vi "Andres  Decoder 3-to-8      Complete.vi"() -> ()   [LabVIEW 2013]
panel:
  out "Boolean 7":bool
  out "Boolean 6":bool
  out "Boolean 5":bool
  out "Boolean 4":bool
  out "Boolean 3":bool
  out "Boolean 2":bool
  out "Boolean 1":bool
  out "Boolean 0":bool
  in  "Digital 2":bool
  in  "Digital 0":bool
  in  "Digital 1":bool
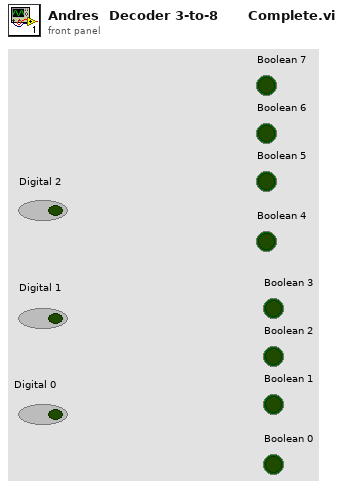
[diagram p1: front panel]
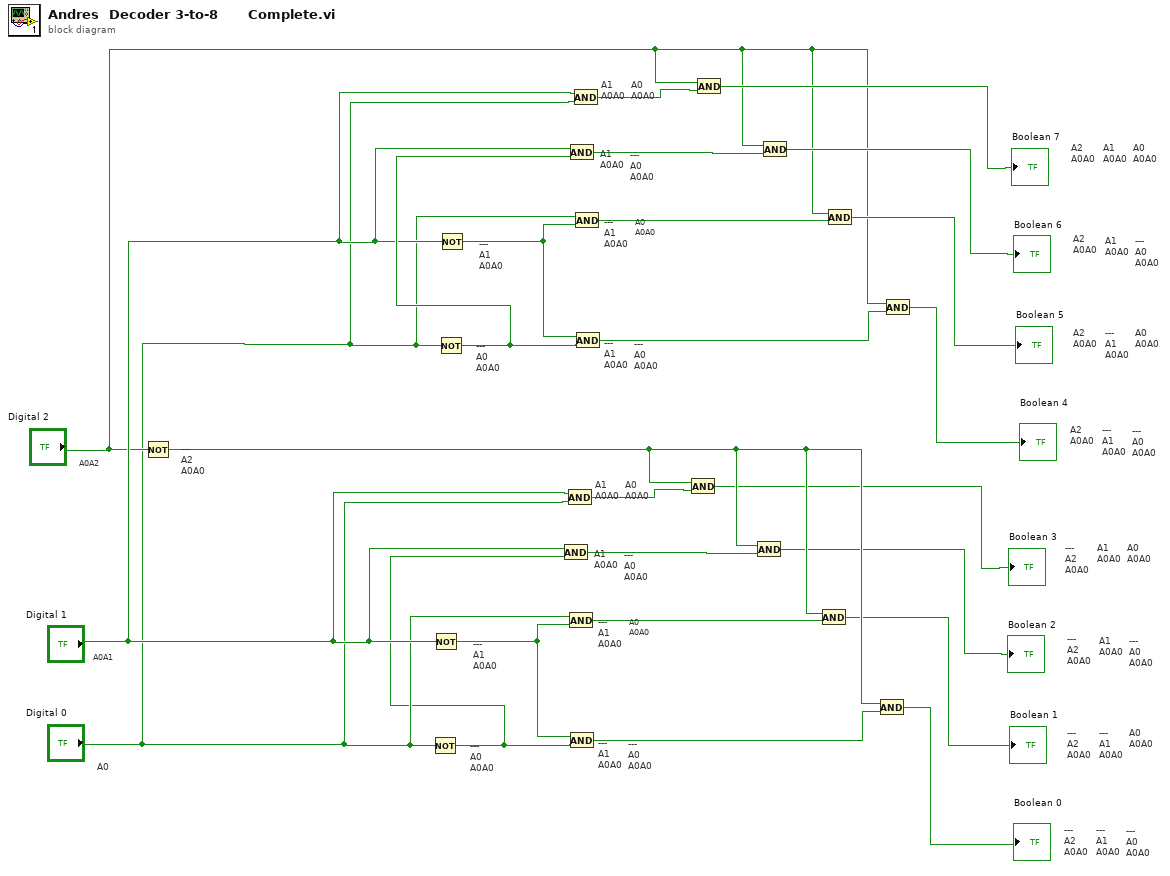
[diagram p0: block diagram]
diagram:
  # "A1\nA0A0"
  # "A0\nA0A0"
  # "---\nA2\nA0A0"
  # "A1\nA0A0"
  # "A0\nA0A0"
  # "A1\nA0A0"
  # "---\nA0\nA0A0"
  # "---\nA2\nA0A0"
  # "A1\nA0A0"
  # "---\nA0\nA0A0"
  # "---\nA1\nA0A0"
  # "A0\nA0A0"
  # "---\nA2\nA0A0"
  # "---\nA1\nA0A0"
  # "A0\nA0A0"
  # "---\nA2\nA0A0"
  # "---\nA1\nA0A0"
  # "---\nA0\nA0A0"
  # "---\nA1\nA0A0"
  # "---\nA0\nA0A0"
  # "---\nA1\nA0A0"
  # "---\nA0\nA0A0"
  # "A1\nA0A0"
  # "A0\nA0A0"
  # "A2\nA0A0"
  # "A1\nA0A0"
  # "A0\nA0A0"
  # "A1\nA0A0"
  # "---\nA0\nA0A0"
  # "A2\nA0A0"
  # "A1\nA0A0"
  # "---\nA0\nA0A0"
  # "---\nA1\nA0A0"
  # "A0\nA0A0"
  # "A2\nA0A0"
  # "---\nA1\nA0A0"
  # "A0\nA0A0"
  # "A2\nA0A0"
  # "---\nA1\nA0A0"
  # "---\nA0\nA0A0"
  # "---\nA1\nA0A0"
  # "---\nA0\nA0A0"
  # "---\nA1\nA0A0"
  # "---\nA0\nA0A0"
  # "A0A1"
  # "A0"
  # "---\nA2\nA0A0"
  # "A0A2"
  n1 = Not(x="Digital 2") -> (.not. x?=w24:bool)
  n2 = Not(x="Digital 0") -> (.not. x?=w5:bool)
  n3 = Not(x="Digital 1") -> (.not. x?=w8:bool)
  n4 = Not(x="Digital 0") -> (.not. x?=w19:bool)
  n5 = Not(x="Digital 1") -> (.not. x?=w22:bool)
  n6 = And(x="Digital 1", y=w5) -> (x .and. y?=w4:bool)
  n7 = And(x="Digital 1", y="Digital 0") -> (x .and. y?=w2:bool)
  n8 = And(x="Digital 0", y=w8) -> (x .and. y?=w7:bool)
  n9 = And(x="Digital 1", y=w19) -> (x .and. y?=w18:bool)
  n10 = And(x=w8, y=w5) -> (x .and. y?=w10:bool)
  n11 = And(x="Digital 1", y="Digital 0") -> (x .and. y?=w16:bool)
  n12 = And(x="Digital 0", y=w22) -> (x .and. y?=w21:bool)
  n13 = And(x=w22, y=w19) -> (x .and. y?=w23:bool)
  n14 = And(x=w24, y=w2) -> (x .and. y?=→"Boolean 3":bool)
  n15 = And(x="Digital 2", y=w16) -> (x .and. y?=→"Boolean 7":bool)
  n16 = And(x=w24, y=w4) -> (x .and. y?=→"Boolean 2":bool)
  n17 = And(x="Digital 2", y=w18) -> (x .and. y?=→"Boolean 6":bool)
  n18 = And(x=w24, y=w7) -> (x .and. y?=→"Boolean 1":bool)
  n19 = And(x="Digital 2", y=w21) -> (x .and. y?=→"Boolean 5":bool)
  n20 = And(x=w24, y=w10) -> (x .and. y?=→"Boolean 0":bool)
  n21 = And(x="Digital 2", y=w23) -> (x .and. y?=→"Boolean 4":bool)
